vi "testDatapass.vi"() -> ()   [LabVIEW 2015]
uses:
  Kobuki Bumps and WheelDrops.ctl
  Kobuki Buttons.ctl
  Charging Sources Available.ctl
  KobukiSensors.ctl
  CyberSim/autograder/feedbackMode.ctl
  CyberSim interface/Simulation Configuration.ctl
  <instrlib>/DC Motor Controller/HAIOL/DC Motor Controller.lvclass
  CyberSim/Multi Bot Code/RobotData.ctl
  CyberSim/simulation/Simulator.ctl
panel:
  out "leftWheelSpeed":i16
  out "rightWheelSpeed":i16
  in  "Kobuki Sensors":T1={"Bumps + Wheel Drops"={"Wheeldrop Left"=FALSE, "Wheeldrop Right"=FALSE, "Bump Left"=FALSE, "Bump Center"=FALSE, "Bump Right"=FALSE}, "Cliff Left"=FALSE, "Cliff Center"=FALSE, "Cliff Right"=FALSE, "Cliff Left Signal"=65413, "Cliff Center Signal"=65302, "Cliff Right Signal"=64969, "Buttons"={"B0"=FALSE, "B1"=FALSE, "B2"=FALSE}, "Left Wheel Encoder (ticks)"=0, "Right Wheel Encoder (ticks) "=0, "Right Wheel Current (x10mA)"=0, "Left  Wheel Current  (x10mA)"=0, "TimeStamp"=0, "Song Playing"=FALSE, "Song Number"=0, "Voltage (mV)"=0, "Current (mA)"=0, "Battery Temperature (deg C)"=0, "Battery Charge (mAh)"=0, "Battery Capacity (mAh)"=0, "Charging Sources"={"Internal Charger"=FALSE, "Home Base"=FALSE}, "Angle( of 100deg)"=0, "Angle Rate( of 100 deg/sec)"=0}
  out "error out":errorcluster
  out "simulator":T5={"configuration"={"maxTime"=5.0, "enableVisualization"=TRUE, "Environment Definition"=path "simulation configuration.ini", "Record Location"=path "Simulation Record.xml", "autograde?"=TRUE, "interactive?"=FALSE, "Feedback Mode"=enum."debug navigation", "Robot State Charts"=[path "C:/Users/blueuser/Desktop/Robo Sim Berkley/cpsgrader-release-0.4/Simulators/EECS149lab/src/LabVIEW/statechart/Simulation Statechart.vi"], "statechart"=path "C:/Users/blueuser/Desktop/Robo Sim Berkley/cpsgrader-release-0.4/Simulators/EECS149lab/src/LabVIEW/statechart/Simulation Statechart.vi"}, "Statechart\ndisplay"=refnum, "first step?"=FALSE, "Robots Simulation Statecharts"=[], "Robots"=[]}
  # "Electrical: charging, battery, OI mode"
  # "Sensors: bump, cliff, button, wheel drop, wall, virtual wall"
  # "Motors:"
  # "Song"
  # "Inertia"
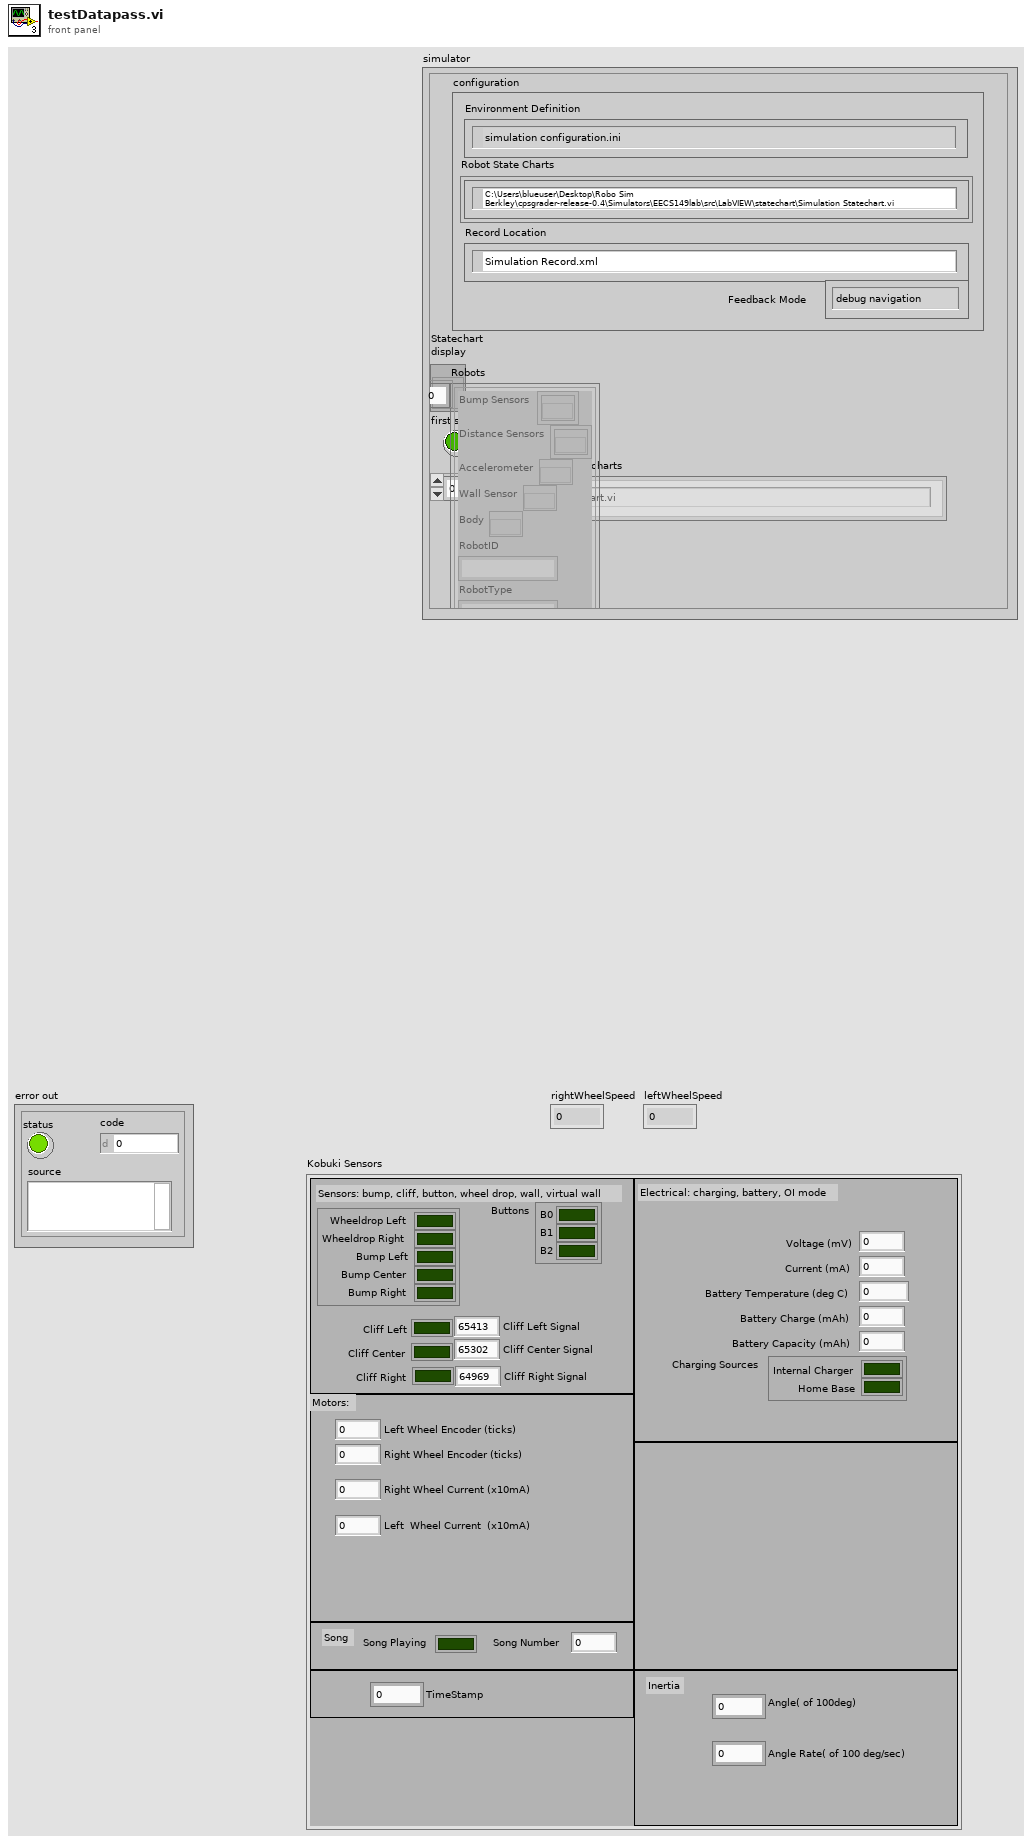
[diagram p1: front panel]
types:
  T1 = typedef "KobukiSensors.ctl" = cluster{"Bumps + Wheel Drops":T2, "Cliff Left":bool, "Cliff Center":bool, "Cliff Right":bool, "Cliff Left Signal":u16, "Cliff Center Signal":u16, "Cliff Right Signal":u16, "Buttons":T3, "Left Wheel Encoder (ticks)":u16, "Right Wheel Encoder (ticks) ":u16, "Right Wheel Current (x10mA)":i16, "Left  Wheel Current  (x10mA)":i16, "TimeStamp":u16, "Song Playing":bool, "Song Number":u8, "Voltage (mV)":i16, "Current (mA)":i16, "Battery Temperature (deg C)":i16, "Battery Charge (mAh)":i16, "Battery Capacity (mAh)":i16, "Charging Sources":T4, "Angle( of 100deg)":i16, "Angle Rate( of 100 deg/sec)":i16}
  T2 = typedef "Kobuki Bumps and WheelDrops.ctl" = cluster{"Wheeldrop Left":bool, "Wheeldrop Right":bool, "Bump Left":bool, "Bump Center":bool, "Bump Right":bool}
  T3 = typedef "Kobuki Buttons.ctl" = cluster{"B0":bool, "B1":bool, "B2":bool}
  T4 = typedef "Charging Sources Available.ctl" = cluster{"Internal Charger":bool, "Home Base":bool}
  T5 = typedef "Simulator.ctl" = cluster{"configuration":T6, "Statechart\ndisplay":refnum<vi>, "first step?":bool, "Robots Simulation Statecharts":path[], "Robots":T8[]}
  T6 = typedef "Simulation Configuration.ctl" = cluster{"maxTime":sgl, "enableVisualization":bool, "Environment Definition":path, "Record Location":path, "autograde?":bool, "interactive?":bool, "Feedback Mode":T7, "Robot State Charts":path[], "statechart":path}
  T7 = typedef "feedbackMode.ctl" = enum32{"debug navigation", "debug hill climb", "autograde navigation", "autograde hill climb"}
  T8 = typedef "RobotData.ctl" = cluster{"Bump Sensors":refnum<k20>[], "Distance Sensors":refnum<k20>[], "Accelerometer":refnum<k20>, "Wall Sensor":refnum<k20>, "Body":refnum<k20>, "RobotID":string, "RobotType":string, "Left Motor":refnum<class "DC Motor Controller.lvclass">, "Right Motor":refnum<class "DC Motor Controller.lvclass">}
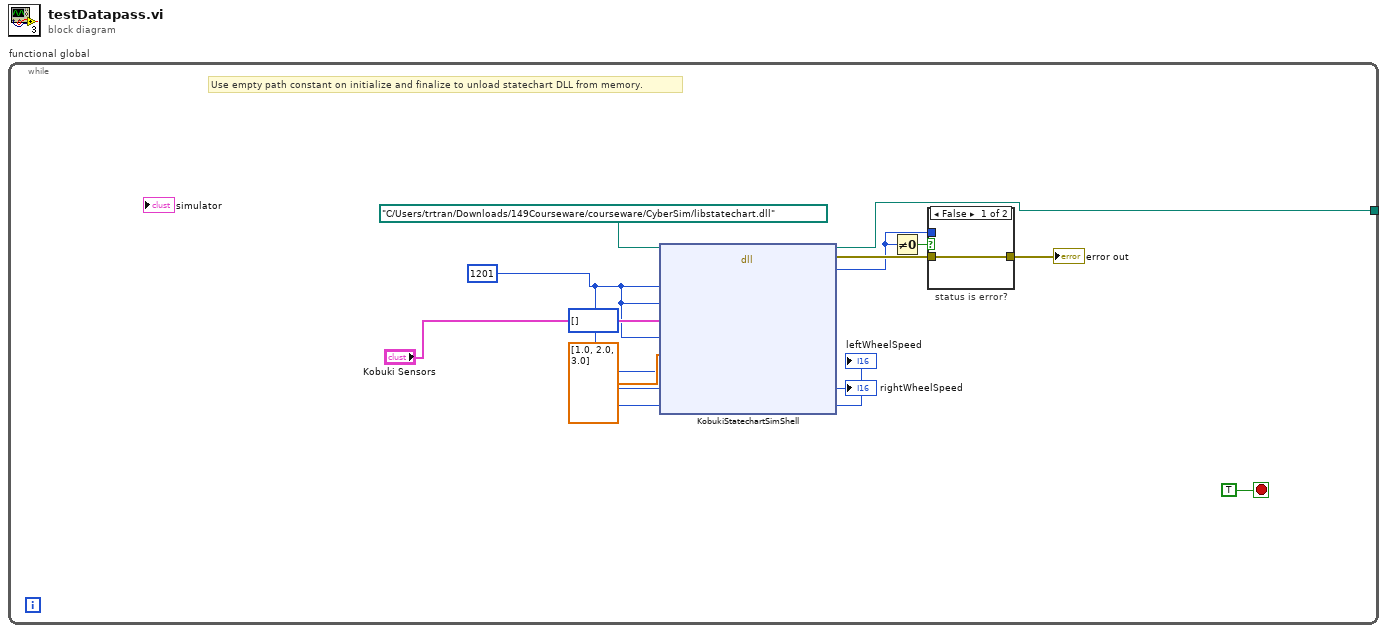
[diagram p0: block diagram]
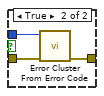
[diagram p2: hidden frame]
diagram:
  n1 = while "functional global" {
    tunnel: [w3] -> _
    stop <- TRUE stop-if-true
    (unwired) u8[] [] ("sensorStream")
    w5 = 1201 ("netDistance")
    # "Use empty path constant on initialize and finalize to unload statechart DLL from memory."
    n2 = dll-call lib="D:/Users/jjensen/workspace/Simulated iRobot Navigation/Release/libSimulated iRobot Navigation.dll" fn="KobukiStatechartSimShell"(path in=path "C:/Users/trtran/Downloads/149Courseware/courseware/CyberSim/libstatechart.dll", "netDistance"=w5, "netAngle"=w5, "sensors"="Kobuki Sensors", "sensorStreamSize"=w5, "accelAxes"=dbl[] [1.0, 2.0, 3.0], "accelAxesSize"=w5, "rightWheelSpeed"=w5, "leftWheelSpeed"=w5) -> (path out=w3:path, error out=w9:errorcluster, "status"=w8:i32, "rightWheelSpeed"=→"rightWheelSpeed":i16, "leftWheelSpeed"=→"leftWheelSpeed":i16)  [unwired: 8 in]
    n3 = Not Equal To 0?(x=w8) -> (x != 0?=w11:bool)
    n4 = case "status is error?" shown="False" w11 {
      tunnel: w8 -> [_ w16]
      tunnel: w9 -> [w13 w15]
      tunnel: [w13 w14] -> w10
      frame False {
      }
      frame True {
        n5 = call <vilib>:"Error Cluster From Error Code.vi"("error in (no error)"=w15, "error code (0)"=w16) -> ("error out"=w14:errorcluster)  [unwired: 7 in]
      }
    }
    "error out" <- w10
  }
